vi "Instrument Status Checking.vi"(8 "error in (no error)":errorcluster, 9 "Status Checking (On)":bool=TRUE, 11 "VISA resource name":refnum<visa-resource-name>) -> (0 "error out":errorcluster, 3 "VISA resource name out":refnum<visa-resource-name>)   [LabVIEW 2015, in "Rohde&Schwarz CMXP NR FR2 Measurement.lvlib"]
doc: "This VI switches state checking of the instrument driver (*STB? query bit 2). Subsequently, all the driver VIs are using the state checking to immediately react on error that might have occured. We recommend to keep the state checking ON all the time. Switch it OFF only in rare cases when you require maximum speed.\nThe default state after initializing the session is <b>ON</b>."
uses:
  <instrlib>/Rohde&Schwarz CMXP NR FR2 Measurement/Rohde&Schwarz CMXP NR FR2 Measurement.lvlib
  <instrlib>/Rohde&Schwarz CMXP NR FR2 Measurement/Private/rsidr_core.llb/type_Session_Parameter_boolean.ctl
  <instrlib>/Rohde&Schwarz CMXP NR FR2 Measurement/Private/rsidr_core.llb/rsidr_core.lvlib
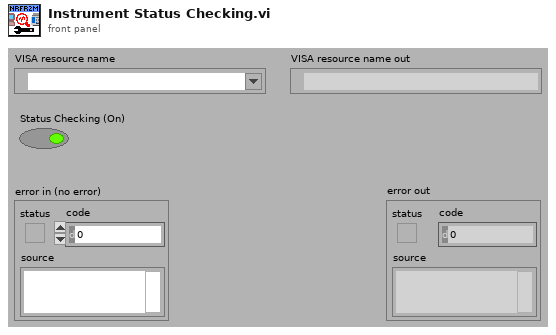
[diagram p1: front panel]
types:
  T1 = typedef "Rohde&Schwarz CMXP NR FR2 Measurement.lvlib/rsidr_core.lvlib/type_Session_Parameter_boolean.ctl" = enum16{"Simulate", "Query Instr Status", "Check Range", "Check Options", "Add LF to Write", "Duplicate Session", "Fast Sweep", "Logging"}
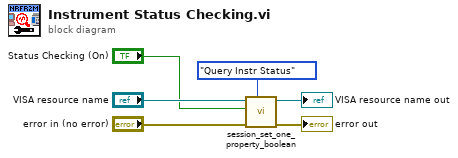
[diagram p0: block diagram]
diagram:
  n1 = call <instrlib>:"session_set_one_property_boolean.vi"("Session Parameter boolean"=type_Session_Parameter_boolean."Query Instr Status", "error in"="error in (no error)", "boolean value in"="Status Checking (On)", "VISA resource name"="VISA resource name") -> ("error out"=→"error out":errorcluster, "VISA resource name out"=→"VISA resource name out":refnum<visa-resource-name>)  [unwired: 5 in, 1 out]
